vi "Test Find Tests From lvlib.vi"(8 "error in (no error)":errorcluster, 11 "Test Case In":refnum<class "Test FInder Test.lvclass">) -> (0 "error out":errorcluster, 3 "Test Case Out":refnum<class "Test FInder Test.lvclass">)   [LabVIEW 2020, in "Test FInder Test.lvclass"]
uses:
  Test FInder Test.lvclass
  C:/Program Files (x86)/National Instruments/LabVIEW 2020/vi.lib/Astemes/LUnit/Test Case.lvclass
  <vilib>/Astemes/LUnit/Test Case.lvclass/Test Case.ctl
  <vilib>/Astemes/LUnit/Palette/Fail.vi
  <vilib>/Astemes/LUnit/Palette/Pass.vi
  <vilib>/Astemes/LUnit/Set Assertion Type.vi
  <vilib>/Astemes/LUnit/Add test result.vi
  <vilib>/Astemes/LUnit/LUnit Record Assertion Result.vi
  <vilib>/Astemes/LUnit/LUnit Aggregate Assertion Results.vi
  <vilib>/Astemes/LUnit/Method Result/LUnit Merge Status.vi
  <vilib>/Astemes/LUnit/LUnit Concatenate result strings.vi
  source/Core/Runnable/Runnable.lvclass
  source/Framework/Test Finder/Test Finder.lvclass
  <vilib>/Astemes/LUnit/Test Case.lvclass
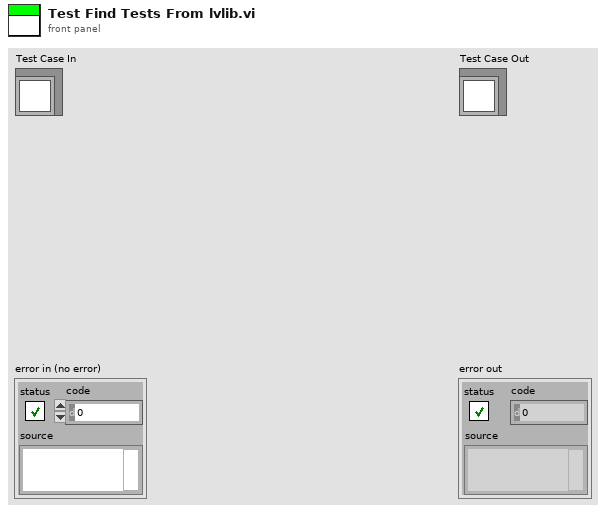
[diagram p1: front panel]
types:
  T1 = typedef "Result.lvlib/Result.ctl" = cluster{"Name":string, "Message":string, "Description":string, "Status":T2, "Result Type":T3, "Execution Time":dbl}
  T2 = typedef "Result.lvlib/Status.ctl" = enum16{"", "Passed", "Failed", "Error", "Skipped", "Setup Error", "Broken", "Teardown Error"}
  T3 = typedef "Result.lvlib/Type.ctl" = enum16{"Method", "Case", "Suite", "Pass", "Fail", "Skip", "Pass if", "Fail if", "Pass if Error", "Fail if Error", "Pass if Equal", "Fail if Equal"}
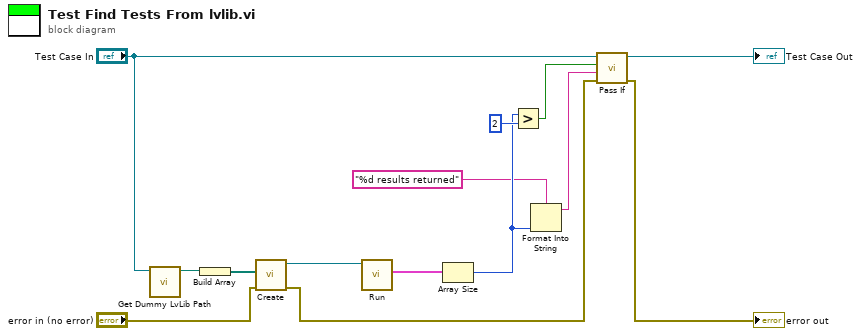
[diagram p0: block diagram]
diagram:
  n1 = call "Get Dummy LvLib Path.vi"("LUnit Test Suite Tests in"="Test Case In") -> ("appended path"=w11:path)  [unwired: 10 in]
  n2 = Build Array(w11) -> (w10:path[])
  n3 = call "Create.vi"("error in (no error)"="error in (no error)", "File Paths"=w10) -> ("error out"=w12:errorcluster, "LUnit Test Suite V2.lvclass"=w9:refnum<class "Runnable.lvclass">)  [unwired: 8 in]
  n4 = call-dynamic "Run.vi"("Runnable In"=w9) -> ("Results"=w8:T1[])  [unwired: 9 in, 1 out]
  n5 = Array Size(array=w8) -> (size(s)=w3:i32)
  n6 = Greater?(x=w3, y=2) -> (0:w4:bool)
  n7 = Format Into String(format string="%d results returned", w3) -> (resulting string=w1:string)  [unwired: 2 in, 1 out]
  n8 = call <vilib>:"Pass If.vi"("error in (no error)"=w12, "Message"=w1, "Pass?"=w4, "LUnit Test Case In"="Test Case In") -> ("error out"=→"error out":errorcluster, "LUnit Test Case Out"=→"Test Case Out":refnum<class "Test FInder Test.lvclass">)  [unwired: 6 in]
